vi "Last Conf Load.vi"(8 "error in":errorcluster, 11 "Config Dir":path) -> (0 "error out":errorcluster, 3 "Conf File path":path)   [LabVIEW 2019, in "Generic Test Stand.lvclass"]
uses:
  Generic Test Stand.lvclass
  <vilib>/Utility/config.llb/Read Key (String).vi
  <vilib>/Utility/config.llb/NI_LVConfig.lvlib
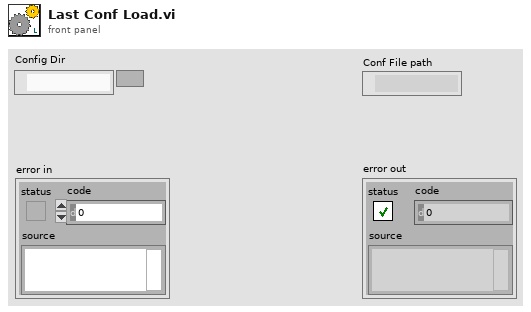
[diagram p1: front panel]
types:
  T1 = typedef "NI_LVConfig.lvlib/Config Data RefNum.ctl" = refnum<k1>
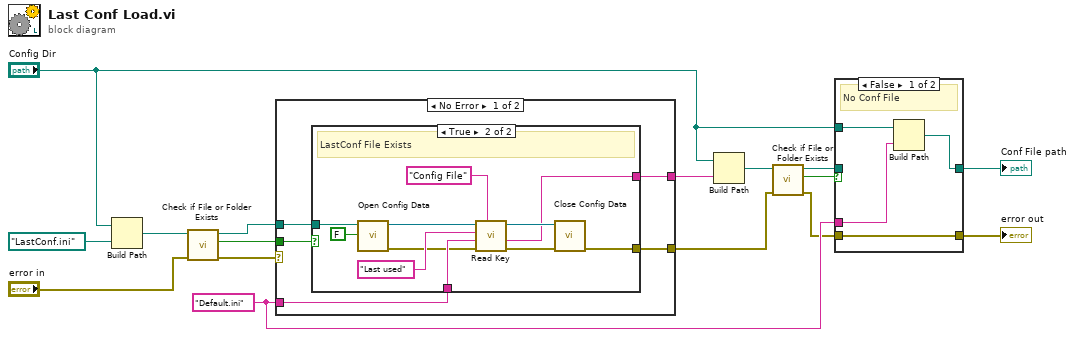
[diagram p0: block diagram]
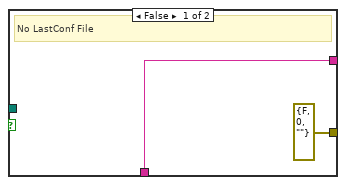
[diagram p3: hidden frame]
diagram:
  w6 = "Default.ini"
  n1 = Build Path(base path="Config Dir", name or relative path=path "LastConf.ini") -> (appended path=w15:path)
  n2 = call <vilib>:"Check if File or Folder Exists.vi"("error in (no error)"="error in", "path"=w15) -> ("error out"=w14:errorcluster, "file or folder exists?"=w13:bool, "dup path"=w12:path)  [unwired: 7 in]
  n3 = case shown="No Error" w14 {
    selector: w14 -> [_ w36]
    tunnel: [w19 w36] -> w10
    tunnel: w13 -> [w21 _]
    tunnel: w12 -> [w20 _]
    tunnel: w6 -> [w18 w35]
    tunnel: [w17 w35] -> w4
    frame No Error {
      n4 = case shown="True" w21 {
        tunnel: w20 -> [_ w34]
        tunnel: w18 -> [w22 w29]
        tunnel: [errorcluster {"status"=FALSE, "code"=0, "source"=""} ("error out") w25] -> w19
        tunnel: [w22 w24] -> w17
        frame False {
          # "No LastConf File"
        }
        frame True {
          # "LastConf File Exists"
          n5 = call <vilib>:"Open Config Data.vi"("create file if necessary (T)"=FALSE, "configuration file path"=w34) -> ("error out"=w28:errorcluster, "refnum"=w32:T1)  [unwired: 7 in, 1 out]
          n6 = call-poly <vilib>:"Read Key.vi"("section"="Config File", "error in (no error)"=w28, "default value"=w29, "key"="Last used", "refnum"=w32) -> ("error out"=w27:errorcluster, "value"=w24:string, "refnum out"=w26:T1)  [unwired: 3 in, 1 out]
          n7 = call <vilib>:"Close Config Data.vi"("error in (no error)"=w27, "refnum"=w26) -> ("error out"=w25:errorcluster)  [unwired: 8 in, 1 out]
        }
      }
    }
    frame Error {
    }
  }
  n8 = Build Path(base path="Config Dir", name or relative path=w4) -> (appended path=w11:path)
  n9 = call <vilib>:"Check if File or Folder Exists.vi"("error in (no error)"=w10, "path"=w11) -> ("error out"=w2:errorcluster, "file or folder exists?"=w9:bool, "dup path"=w8:path)  [unwired: 7 in]
  n10 = case shown="False" w9 {
    tunnel: w8 -> [_ w42]
    tunnel: "Config Dir" -> [w40 _]
    tunnel: w6 -> [w37 _]
    tunnel: [w39 w42] -> w5
    tunnel: [w38 w41] -> w3
    tunnel: w2 -> [w38 w41]
    frame False {
      # "No Conf File"
      n11 = Build Path(base path=w40, name or relative path=w37) -> (appended path=w39:path)
    }
    frame True {
      # "Conf File Exists"
    }
  }
  "error out" <- w3
  "Conf File path" <- w5
